vi "fgv.vi"() -> ()   [LabVIEW 2020]
panel:
  in  "Enum":enum16{"increase", "decrase", "reset", ""}(ring)
  out "Numeric":dbl
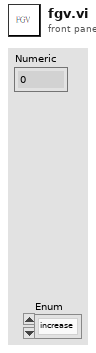
[diagram p1: front panel]
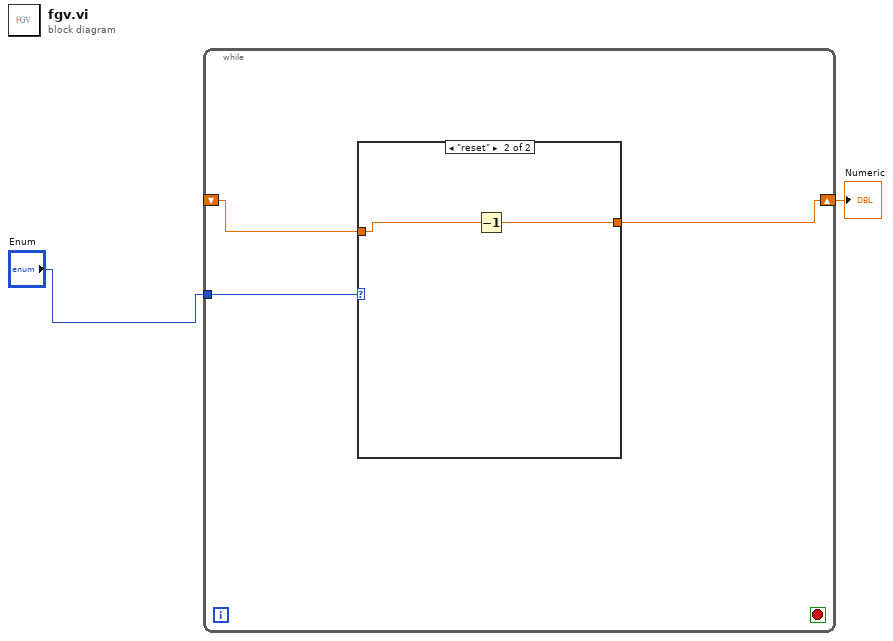
[diagram p0: block diagram]
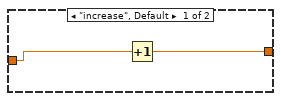
[diagram p2: hidden frame]
diagram:
  n1 = while {
    tunnel: "Enum" -> [w3]
    shift-right: [w4] -> w2
    shift-left: _ -> [w5]
    stop <- _ stop-if-true
    n2 = case shown="\"reset\"" w3 {
      tunnel: w5 -> [w7 w9]
      tunnel: [w6 w8] -> w4
      frame "increase", Default {
        n3 = Increment(x=w7) -> (x+1=w6:dbl)
      }
      frame "reset" {
        n4 = Decrement(x=w9) -> (x-1=w8:dbl)
      }
    }
  }
  "Numeric" <- w2
